vi "Read Image Resolution.vi"(8 "error in (no error)":errorcluster, 11 "Camera in":refnum<class "Camera.lvclass">) -> (0 "error out":errorcluster, 2 "Image Resolution":T1, 3 "Camera out":refnum<class "Camera.lvclass">)   [LabVIEW 2018, in "Camera.lvlib" / "Camera.lvclass"]
uses:
  Camera.lvclass
  Custom Controls/Image Resolution.ctl
  Camera.lvclass/Camera.ctl
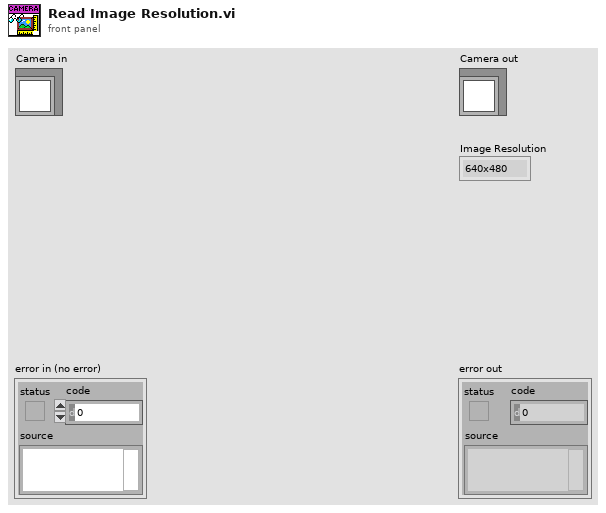
[diagram p1: front panel]
types:
  T1 = typedef "Camera.lvlib/Camera.lvclass/Image Resolution.ctl" = enum16{"640x480", "1024x768", "1280x720", "1280x1024", "1600x1200", "1920x1080", "1920x1200"}
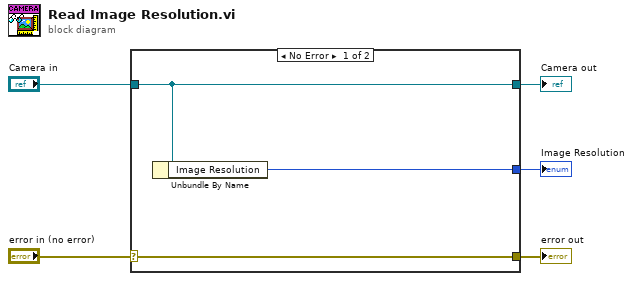
[diagram p0: block diagram]
diagram:
  n1 = case shown="No Error" "error in (no error)" {
    selector: "error in (no error)" -> [w8 w9]
    tunnel: [w8 w9] -> w4
    tunnel: [w7 w10] -> w2
    tunnel: "Camera in" -> [w7 w10]
    tunnel: [w6 _] -> w1
    frame No Error {
      n2 = Unbundle By Name(w7) -> ("Image Resolution"=w6:T1)
    }
    frame Error {
    }
  }
  "error out" <- w4
  "Camera out" <- w2
  "Image Resolution" <- w1
